vi "Get Panel Ref.vi"(8 "error in (no error)":errorcluster, 11 "Panel in":refnum<class "Panel.lvclass">) -> (0 "error out":errorcluster, 2 "Panel Ref":refnum<vi>, 3 "Panel out":refnum<class "Panel.lvclass">)   [LabVIEW 2020, in "OOPanel.lvlib" / "Panel.lvclass"]
uses:
  Panel.lvclass
  Visibility State.ctl
  Panel.lvclass/Panel.ctl
  <vilib>/Utility/error.llb/Error Cluster From Error Code.vi
  <vilib>/ErrorRing/Error Ring.xnode
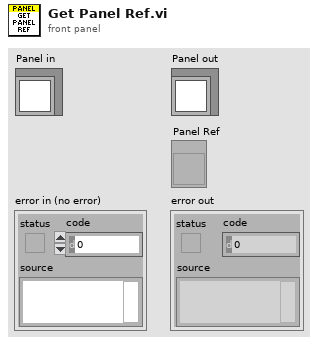
[diagram p1: front panel]
types:
  T1 = typedef "OOPanel.lvlib/Panel.lvclass/Visibility State.ctl" = enum16{"Idle", "Closed", "Hidden", "Visible", "Subpanel"}
  T2 = typedef "OOPanel.lvlib/Panel.lvclass/Ref Data.ctl" = cluster{"Panel Events":T3, "Panel Ref":refnum<vi>, "SubPanel":refnum<vi>, "Close":bool, "Running":bool, "State":T1}
  T3 = typedef "OOPanel.lvlib/Panel.lvclass/Panel Events.ctl" = cluster{"Visbility":refnum<user-event>, "Close":refnum<user-event>}
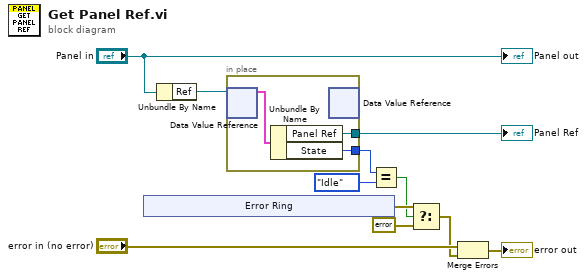
[diagram p0: block diagram]
diagram:
  n1 = xnode "Error Ring"() -> ("error out"=w6:errorcluster)
  n2 = Unbundle By Name("Panel in") -> ("Ref"=w10:refnum<data-value>)
  n3 = in-place {
    in-place-border: [w13] -> w8
    in-place-border: [w12] -> w3
    n4 = in-place-dvr #1(w10) -> (w14:T2)  [unwired: 1 out]
    n5 = Unbundle By Name(w14) -> ("Panel Ref"=w13:refnum<vi>, "State"=w12:T1)
    n6 = in-place-dvr #1() -> ()  [unwired: 1 in, 2 out]
  }
  "Panel Ref" <- w8
  n7 = Equal?(x=w3, y=Visibility_State."Idle") -> (x = y?=w4:bool)
  n8 = Select(t=w6, s=w4, f=errorcluster {"status"=FALSE, "code"=0, "source"=""}) -> (s? t:f=w1:errorcluster)
  n9 = Merge Errors("error in (no error)", w1) -> (→"error out":errorcluster)
  "Panel out" <- "Panel in"
